vi "ThetaPhi2Dir.vi"(10 "Phi":dbl, 11 "Theta":dbl) -> (3 "Dir":dbl[](array[numeric]))   [LabVIEW 2014]
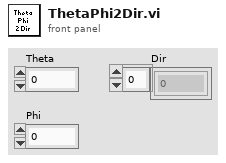
[diagram p1: front panel]
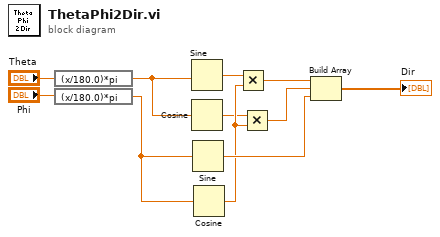
[diagram p0: block diagram]
diagram:
  n1 = expression code="(x/180.0)*pi" ("degrees to radians")("Theta") -> (w9:dbl)
  n2 = expression code="(x/180.0)*pi" ("degrees to radians")("Phi") -> (w11:dbl)
  n3 = Sine(x=w9) -> (sin(x)=w3:dbl)
  n4 = Cosine(x=w9) -> (cos(x)=w4:dbl)
  n5 = Sine(x=w11) -> (sin(x)=w7:dbl)
  n6 = Cosine(x=w11) -> (cos(x)=w5:dbl)
  n7 = Multiply(x=w3, y=w5) -> (x*y=w2:dbl)
  n8 = Multiply(x=w4, y=w5) -> (x*y=w6:dbl)
  n9 = Build Array(w2, w6, w7) -> (→"Dir":dbl[])
